vi "example_02_visualization.vi"() -> ()   [LabVIEW 2015, in "lv-calibration.lvlib"]
uses:
  lv-calibration.lvlib
  public/_controls/configuration.ctl
  public/_controls/type.ctl
  public/_controls/point.ctl
  <userlib>/antonio-alexander/lv-graph/public/advanced/build_graph-multiple_axis.vi
  <userlib>/antonio-alexander/lv-graph/lv-graph.lvlib
panel:
  in  "configuration":T1={"tag_name"="tag-001", "type"="slope_intercept", "zero"=0.0, "formula"="", "points"=[{"x"=10.0, "y"=100.0}]}
  out "graph":cluster{dbl[], dbl[]}[](graph)
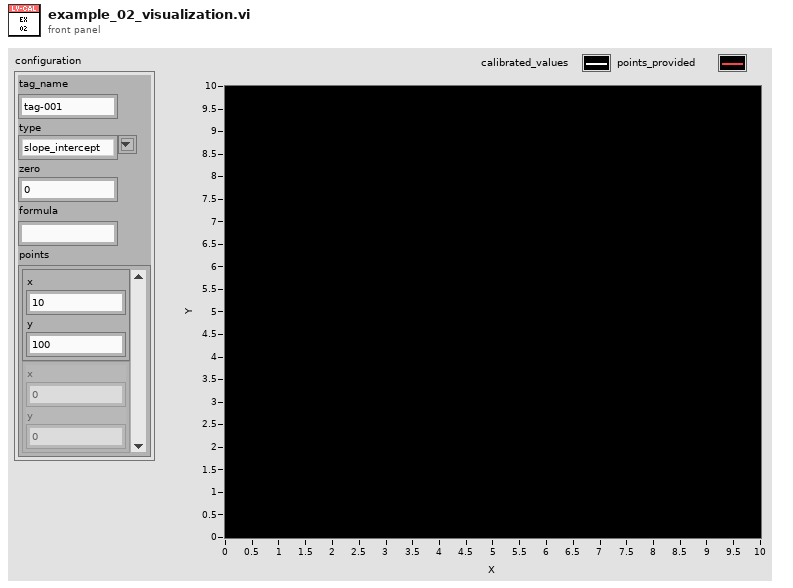
[diagram p1: front panel]
types:
  T1 = typedef "lv-calibration.lvlib/configuration.ctl" = cluster{"tag_name":string, "type":T2, "zero":dbl, "formula":string, "points":T3[]}
  T2 = typedef "lv-calibration.lvlib/type.ctl" = string
  T3 = typedef "lv-calibration.lvlib/point.ctl" = cluster{"x":dbl, "y":dbl}
  T4 = typedef "lv-calibration.lvlib/runtime.ctl" = cluster{"tag_name":string, "type":T2, "offset":dbl, "slope":dbl, "formula":string, "x_points":dbl[], "y_points":dbl[]}
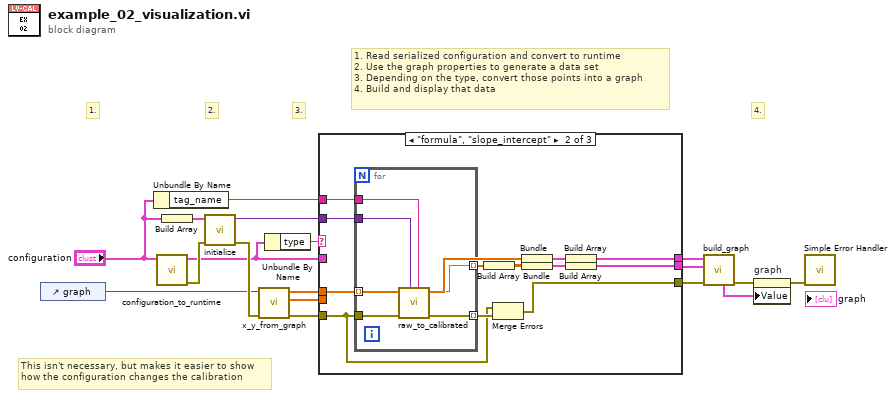
[diagram p0: block diagram]
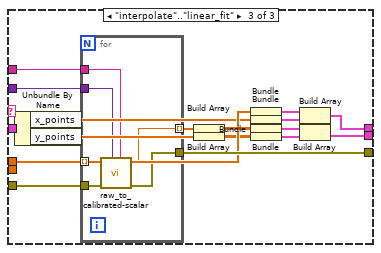
[diagram p3: hidden frame]
diagram:
  # "4."
  # "3."
  # "2."
  # "1."
  # "This isn't necessary, but makes it easier to show\nhow the configuration changes the calibration"
  # "1. Read serialized configuration and convert to runtime\n2. Use the graph properties to generate a data set\n3. Depending on the type, convert those points into a graph\n4. Build and display that data"
  n1 = control-ref of="graph"() -> (w13:refnum<vi>)
  n2 = Unbundle By Name("configuration") -> ("tag_name"=w3:string)
  n3 = call "configuration_to_runtime.vi"("configuration"="configuration") -> ("error out"=w18:errorcluster, "runtime"=w7:T4)  [unwired: 9 in]
  n4 = Build Array("configuration") -> (w6:T1[])
  n5 = call "initialize.vi"("error in (no error)"=w18, "configuration []"=w6) -> ("error out"=w17:errorcluster, "runtime_data"=w4:variant)  [unwired: 8 in]
  n6 = call "x_y_from_graph.vi"("error in (no error)"=w17, "graph_reference"=w13) -> ("error out"=w12:errorcluster, "y []"=w10:dbl[], "x []"=w11:dbl[])  [unwired: 7 in]
  n7 = Unbundle By Name(w7) -> ("type"=w16:T2)
  n8 = case shown="\"formula\", \"slope_intercept\"" w16 {
    tunnel: w7 -> [_ _ w43]
    tunnel: w12 -> [w19 w20 w49]
    tunnel: w11 -> [_ w23 w45]
    tunnel: w10 -> [_ _ _]
    tunnel: [w19 w21 w48] -> w9
    tunnel: [_ w30 w53] -> w8
    tunnel: [_ w28 w51] -> w2
    tunnel: w4 -> [_ w24 w46]
    tunnel: w3 -> [_ w22 w44]
    frame Default {
    }
    frame "formula", "slope_intercept" {
      n9 = for {
        tunnel: [w35] -> w25 mode=indexing
        tunnel: w24 -> [w34]
        tunnel: w20 -> [w37]
        tunnel: [w36] -> w26 mode=indexing
        tunnel: w23 -> [w33] mode=indexing
        tunnel: w22 -> [w32]
        n10 = call-poly "raw_to_calibrated.vi"("tag_name"=w32, "runtime"=w34, "error in (no error)"=w37, "value in"=w33) -> ("error out"=w36:errorcluster, "value out"=w35:dbl)  [unwired: 6 in]
      }
      n11 = Build Array(w25) -> (w27:dbl[][])
      n12 = Merge Errors(w20, w26) -> (w21:errorcluster)
      n13 = Bundle("x []"=w23) -> (w31:cluster{"x []":dbl[]})  [unwired: 1 in]
      n14 = Bundle(w27) -> (w29:cluster{dbl[][]})  [unwired: 1 in]
      n15 = Build Array(w31) -> (w30:cluster{"x []":dbl[]}[])
      n16 = Build Array(w29) -> (w28:cluster{dbl[][]}[])
    }
    frame "interpolate".."linear_fit" {
      n17 = Unbundle By Name(w43) -> ("x_points"=w40:dbl[], "y_points"=w39:dbl[])
      n18 = for {
        tunnel: [w58] -> w47 mode=indexing
        tunnel: w46 -> [w57]
        tunnel: w49 -> [w60]
        tunnel: [w59] -> w48
        tunnel: w45 -> [w56] mode=indexing
        tunnel: w44 -> [w55]
        n19 = call "raw_to_calibrated-scalar.vi"("tag_name"=w55, "runtime"=w57, "error in (no error)"=w60, "value in"=w56) -> ("error out"=w59:errorcluster, "value out"=w58:dbl)  [unwired: 6 in]
      }
      n20 = Build Array(w47) -> (w50:dbl[][])
      n21 = Build Array(w39) -> (w42:dbl[][])
      n22 = Bundle("x []"=w45) -> (w54:cluster{"x []":dbl[]})  [unwired: 1 in]
      n23 = Bundle("x_points"=w40) -> (w41:cluster{"x_points":dbl[]})  [unwired: 1 in]
      n24 = Bundle(w50) -> (w52:cluster{dbl[][]})  [unwired: 1 in]
      n25 = Bundle(w42) -> (w38:cluster{dbl[][]})  [unwired: 1 in]
      n26 = Build Array(w54, w41) -> (w53:cluster{"x_points":dbl[]}[])
      n27 = Build Array(w52, w38) -> (w51:cluster{dbl[][]}[])
    }
  }
  n28 = call-poly <userlib>:"build_graph.vi"("error in (no error)"=w9, "y_axis"=w2, "x_axis"=w8) -> ("error out"=w15:errorcluster, "graph_data"=w14:cluster{dbl[], dbl[]}[])  [unwired: 6 in, 1 out]
  n29 = property on="graph" class="XYGraph (strict)"(error in=w15, "Value"=w14) -> (error out=w1:errorcluster)  [unwired: 1 in, 1 out]
  n30 = call <vilib>:"Simple Error Handler.vi"("error in (no error)"=w1) -> ()  [unwired: 4 in, 5 out]
